vi "sub_ReadInput.vi"(8 "error in (no error)":errorcluster, 10 "Dynamic data":T1, 11 "Input parameters":T2={"Measurement type"=enum."Test", "Sensor type"=enum."One channel", "Input file"="", "Output file"="test.txt", "Open after execution?"=FALSE, "Display channel"=0, "Voltage Delay (s)"=0.5, "Switch Delay (s)"=0.01, "VISA resource name source"="", "VISA resource name LCR"="", "Voltage Limit (V)"=1000.0, "Enable Voltage Auto Range (T:Enable)"=TRUE, "Voltage Manual Range (1.0)"=1.0, "Compliance  Level (uA)"=10.0} {"Voltage Limit (V)" format="%#_13g"; "Voltage Delay (s)" format="%#_13g"; "Switch Delay (s)" format="%#_13g"}) -> (0 "error out":errorcluster, 2 "Dynamic data":T1, 3 "Input parameters":T2={"Measurement type"=enum."Test", "Sensor type"=enum."One channel", "Input file"="", "Output file"="test.txt", "Open after execution?"=FALSE, "Display channel"=0, "Voltage Delay (s)"=0.5, "Switch Delay (s)"=0.01, "VISA resource name source"="", "VISA resource name LCR"="", "Voltage Limit (V)"=1000.0, "Enable Voltage Auto Range (T:Enable)"=TRUE, "Voltage Manual Range (1.0)"=1.0, "Compliance  Level (uA)"=10.0} {"Voltage Limit (V)" format="%#_13g"; "Voltage Delay (s)" format="%#_13g"; "Switch Delay (s)" format="%#_13g"})   [LabVIEW 2015]
uses:
  <vilib>/Utility/file.llb/Read Delimited Spreadsheet (DBL).vi
  Input_parameters.ctl
  Dynamic_data.ctl
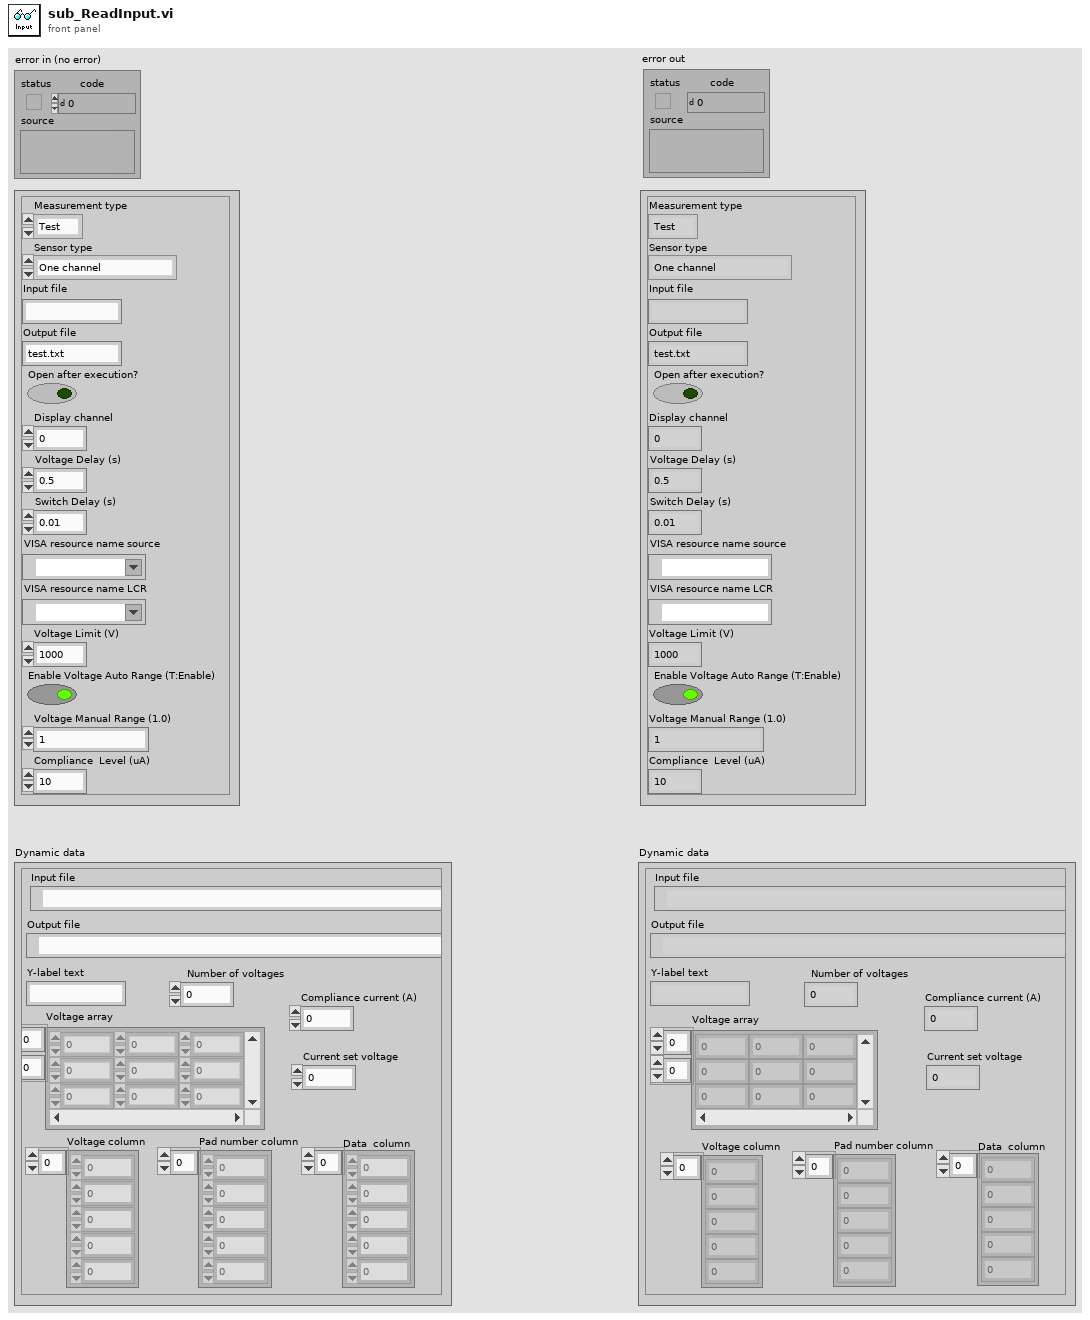
[diagram p1: front panel]
types:
  T1 = typedef "Dynamic_data.ctl" = cluster{"Input file":path, "Output file":path, "Y-label text":string, "Voltage array":dbl[][], "Current set voltage":dbl, "Voltage column":dbl[], "Pad number column":dbl[], "Data  column":dbl[], "Number of voltages":i32, "Compliance current (A)":dbl}
  T2 = typedef "Input_parameters.ctl" = cluster{"Measurement type":enum16{"IV", "CV", "Test"}, "Sensor type":enum16{"6''", "8''", "One channel"}, "Input file":string, "Output file":string, "Open after execution?":bool, "Display channel":i32, "Voltage Delay (s)":dbl, "Switch Delay (s)":dbl, "VISA resource name source":refnum<visa-resource-name>, "VISA resource name LCR":refnum<visa-resource-name>, "Voltage Limit (V)":dbl, "Enable Voltage Auto Range (T:Enable)":bool, "Voltage Manual Range (1.0)":dbl, "Compliance  Level (uA)":dbl}
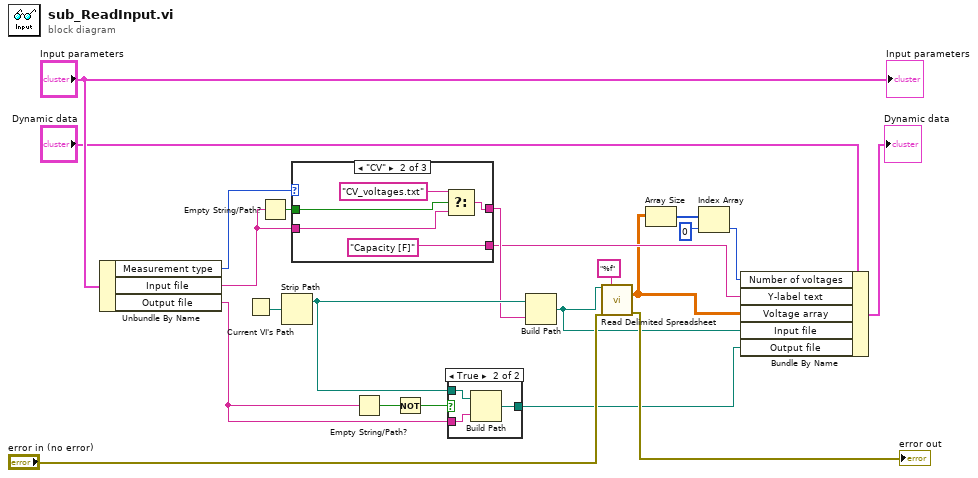
[diagram p0: block diagram]
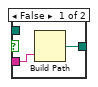
[diagram p2: hidden frame]
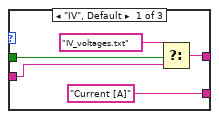
[diagram p3: hidden frame]
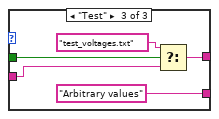
[diagram p4: hidden frame]
diagram:
  n1 = Unbundle By Name("Input parameters") -> ("Measurement type"=w13:enum16{"IV", "CV", "Test"}, "Input file"=w12:string, "Output file"=w15:string)
  n2 = Current VI's Path() -> (path=w21:path)
  n3 = Empty String/Path?(string/path=w12) -> (empty?=w11:bool)
  n4 = Strip Path(path=w21) -> (stripped path=w14:path)  [unwired: 1 out]
  n5 = case shown="\"CV\"" w13 {
    tunnel: ["Current [A]" "Capacity [F]" "Arbitrary values"] -> w6
    tunnel: w12 -> [w23 w29 w34]
    tunnel: w11 -> [w24 w30 w35]
    tunnel: [w26 w28 w33] -> w10
    frame "IV", Default {
      n6 = Select(t="IV_voltages.txt" ("name or relative path"), s=w24, f=w23) -> (s? t:f=w26:string)
    }
    frame "CV" {
      n7 = Select(t="CV_voltages.txt" ("name or relative path"), s=w30, f=w29) -> (s? t:f=w28:string)
    }
    frame "Test" {
      n8 = Select(t="test_voltages.txt" ("name or relative path"), s=w35, f=w34) -> (s? t:f=w33:string)
    }
  }
  n9 = Empty String/Path?(string/path=w15) -> (empty?=w20:bool)
  n10 = Not(x=w20) -> (.not. x?=w19:bool)
  n11 = case shown="True" w19 {
    tunnel: w15 -> [w39 w42]
    tunnel: w14 -> [_ w41]
    tunnel: [w38 w40] -> w7
    frame False {
      n12 = Build Path(name or relative path=w39) -> (appended path=w38:path)  [unwired: 1 in]
    }
    frame True {
      n13 = Build Path(base path=w41, name or relative path=w42) -> (appended path=w40:path)
    }
  }
  n14 = Build Path(base path=w14, name or relative path=w10) -> (appended path=w5:path)
  n15 = call-poly <vilib>:"Read Delimited Spreadsheet.vi"("file path (dialog if empty)"=w5, "format (%.3f)"="%f", "error in (no error)"="error in (no error)") -> ("all rows"=w2:dbl[][], "error out"=→"error out":errorcluster)  [unwired: 7 in, 4 out]
  n16 = Array Size(array=w2) -> (size(s)=w4:i32[])
  n17 = Index Array(array=w4, index=0) -> (element=w1:i32)
  n18 = Bundle By Name(cluster="Dynamic data", "Number of voltages"=w1, "Y-label text"=w6, "Voltage array"=w2, "Input file"=w5, "Output file"=w7) -> (→"Dynamic data":T1)
  "Input parameters" <- "Input parameters"
